vi "Main_capacitor-load.vi"(8 "error in":errorcluster) -> (0 "error out":errorcluster)   [LabVIEW 2019]
uses:
  _ctrl/create-rw-close.ctl
  Register/q-action_reg.ctl
  _ctrl/init-r-stop.ctl
  _ctrl/BP4610_cmd.ctl
  _ctrl/rw.ctl
  _ctrl/DSP_action.ctl
  _ctrl/Testing-info.ctl
  _ctrl/TestType.ctl
  ref_cap_ctrl-ref.ctl
  _ctrl/start.ctl
  common/Global 1.vi
  Devices/NI Board/cDAQ-9476 DO/cnt_Relay.ctl
  Devices/NI Board/cDAQ-9476 DO/cnt_do.ctl
  Devices/NI Board/cDAQ-9269 AO/type_signal.ctl
  Devices/NI Board/cDAQ-9269 AO/AO_q-data.ctl
  sequence_single.ctl
  SubVIs/common/Sample Check.ctl
  Data_cap.ctl
  cap_config.ctl
  Breakdown-Spec.ctl
  _ctrl/Error list.ctl
  _ctrl/DL950_config.ctl
  _ctrl/cDAQ-9269 Config.ctl
  Devices/NI Board/cDAQ-9269 AO/Set_AO_Wave-config.ctl
  Devices/NI Board/cDAQ-9221 AI/Set_NIAI.ctl
  _ctrl/BP4610_config.ctl
  _ctrl/DSP_config.ctl
panel:
  in  "수동_dl950":bool
  in  "수동_6":bool
  out "read_dl950":string
  out "error cluster 2":T1
  in  "Tab main":T2
  out "Relay6 result":T3
  out "Relay5 result":T3
  out "Relay4 result":T3
  out "Relay3 result":T3
  out "Relay2 result":T3
  out "Relay1 result":T3
  out "Graph 6":dbl[](graph)
  out "Graph 5":dbl[](graph)
  out "Graph 4":dbl[](graph)
  out "Graph 3":dbl[](graph)
  out "Graph 2":dbl[](graph)
  out "Graph 1":dbl[](graph)
  out "현재 채널":u8
  out "진행율_채널 %":u8(slide) scale=0.0..100.0
  out "진행율_전체 %":u8(slide) scale=0.0..100.0
  in  "파일 생성 주기[N]":dbl
  in  "저장 경로":path
  in  "시험명":string
  in  "CapTestSpec":T5 {"출력단 특성전류 Irms[mA]  Min" format="%#.2f"; "출력단 특성 전류 Irms[mA]  Max" format="%#.2f"; "출력단 단선 Irms[mA](이하)" format="%#.2f"; "제어단 특성 전류 Irms[mA] Min" format="%#.2f"; "제어단 특성 전류 Irms[mA] Max" format="%#.2f"; "제어단 단선 Irms[mA](이하)" format="%#.2f"}
  in  "CapTestConfig":T6={"출력전압[V]"=0.0, "출력전류[A]"=0.0, "방전 기준[V]"=0.0, "Freq"=0.0, "level[V]"=0.0, "duty"=0.0, "On time[ms]"=0.0, "Record Len"=4, "Time Div"=7, "Repeate"=1, "Test Cycle"=1, "OVP Level"=0.0, "OCP Level"=0.0, "Voltage+[V]"=20.0, "Current+[A]"=5.0, "Voltage-[V]"=-20.0, "Current-[A]"=-5.0} {"Current-[A]" min=-20.0 max=20.0 step=0.001; "Voltage-[V]" min=-115.0 max=115.0 step=0.01; "Current+[A]" min=0.0 max=60.0 step=0.01; "Voltage+[V]" min=0.0 max=120.0 step=0.1; "OCP Level" format="%#_13g"; "OVP Level" format="%#_13g"; "Time Div" items=["10m", "20ms", "50ms", "100ms", "200ms", "500ms", "1s", "2s"]; "Record Len" items=["10k", "25k", "50k", "100k", "250k", "500k", "1M", "2.5M", "5M", "10M", "25M", "50M", "100M", "250M", "500M", "1G", "2G", "4G", "5G", "10G", "20G", "50G"]}
  in  "Tab device":T7(tab)
  in  "DL950_config":T8={"Timeout"=10000, "Time Div"=19, "Acq Mode"=0, "Record Len"=5, "Record Num"=0, "Start Point"=0, "End Poin"=60000, "Visa"="TCPIP0::192.168.0.100::inst0::INSTR", "Config Voltage"=[{"Enable"=TRUE, "Ch"=0, "V Div"=12, "Coupling"=1, "Probe"=3, "Act.Items"=FALSE, "items"=[]}, {"Enable"=TRUE, "Ch"=0, "V Div"=12, "Coupling"=1, "Probe"=3, "Act.Items"=FALSE, "items"=[]}], "Trigger on"=FALSE, "Trigger Level"=0.0, "Reset"=FALSE, "Config Temp"=[], "Trig Mode"=1, "Trig Pos"=50.0, "Trigger Slope"=0, "Trigger Source "=1, "Trig Start -5"=-5.0, "End 5"=5.0} {"End 5" format="%.2g"; "Trig Start -5" format="%.2f"; "Trigger Source" items=["", "CH1", "CH2", "CH3", "CH4", "CH5", "CH6", "CH7", "CH8", "CH9", "CH10", "CH11", "CH12", "CH13", "CH14", "CH15", "CH16", "RMATH1", "RMATH2", "RMATH3", "RMATH4", "RMATH5", "RMATH6", "RMATH7", "RMATH8", "RMATH9", "RMATH10", "RMATH11", "RMATH12", "RMATH13", "RMATH14", "RMATH15", "RMATH16"]; "Trigger Slope" items=["Rising", "Falling", "Both"]; "Trig Pos" format="%.1f"; "Trig Mode" items=["Normal", "Auto", "Auto Level", "Single", "Single(N)", "On Start", "No Set"]; "Config Temp"."Type" items=["K", "E", "J", "T", "L", "U", "N", "R", "S", "B", "W", "Au7fe"]; "Config Temp"."Channel" items=["", "CH1", "CH2", "CH3", "CH4", "CH5", "CH6", "CH7", "CH8", "CH9", "CH10", "CH11", "CH12", "CH13", "CH14", "CH15", "CH16"]; "Trigger Level" format="%.3p"; "Config Voltage"."items" items=["Peak to Peak", "Amplitude", "Max", "Min", "High", "Low", "Average", "Middle", "Rms", "Standard Deviation", "+Overshoot", "-Overshoot", "Rise", "Fall", "Frequency", "Period", "+Width", "-Width", "Duty Cycle", "Pulse Count", "Burst1 Width", "Burst2 Width", "Average Frequency", "Average Period", "Int1TY", "Int2TY"]; "Config Voltage"."Probe" items=["1:1", "2:1", "5:1", "10:1", "20:1", "50:1", "100:1", "200:1", "500:1", "1000:1", "2000:1", "5000:1", "10k:1", "20k:1", "50k:1", "0.1A:1V", "0.2A:1V", "0.5A:1V", "1A:1V", "2A:1V", "5A:1V", "10A:1V", "20A:1V", "50A:1V", "100A:1V", "200A:1V", "250A:1V", "400A:1V", "500A:1V", "1kA:1V", "2kA:1V", "5kA:1V", "10kA:1V", "20kA:1V", "50kA:1V", "NoSet"]; "Config Voltage"."Ch" items=["None", "CH1", "CH2", "CH3", "CH4", "CH5", "CH6", "CH7", "CH8", "CH9", "CH10", "CH11", "CH12", "CH13", "CH14", "CH15", "CH16", "MATH1", "MATH2", "MATH3", "MATH4", "MATH5", "MATH6", "MATH7", "MATH8", "EVENT"]; "Config Voltage"."Coupling" items=["AC", "DC", "Ground", "AC-RMS", "DC-RMS"]; "Config Voltage"."V Div" items=["0.1m", "0.2m", "0.5m", "1m", "2m", "5m", "10m", "20m", "50m", "100m", "200m", "500m", "1", "2", "4", "5", "8", "10", "20", "40", "50", "80", "100", "200", "400", "500", "800", "1k", "2k", "4k", "5k", "8k", "10k", "20k", "25k", "50k", "100k", "250k", "500k", "1000k"]; "Record Len" items=["10k", "25k", "50k", "100k", "250k", "500k", "1M", "2.5M", "5M", "10M", "25M", "50M", "100M", "250M", "500M", "1G", "2G", "4G", "5G", "10G", "20G", "50G"]; "Acq Mode" items=["Normal", "Average", "Envelope"]; "Time Div" items=["100ns", "200ns", "500ns", "1us", "2us", "5us", "10us", "20us", "50us", "100us", "200us", "500us", "1ms", "2ms", "5ms", "10ms", "20ms", "50ms", "100ms", "200ms", "500ms", "1s", "2s", "3s", "4s", "5s", "6s", "10s", "20s", "30s", "1min", "2min", "3min", "4min", "5min", "6min", "10min", "12min", "30min", "1hour", "2hour", "3hour", "4hour", "5hour", "6hour", "8hour", "10hour", "12hour", "1day", "2day", "3day", "4day", "5day"]}
  in  "BP4610 Config":T9={"VISA"="", "Limit-BP"={"Set"=enum."Current", "Voltage+[V]"=20.0, "Current+[A]"=5.0, "Voltage-[V]"=-20.0, "Current-[A]"=-5.0}, "SET BP"={"Set"=enum."FREQ/WAVE", "Operation mode"=0, "Voltage[Vp-p]"=0.0, "Current[Ap-p]"=0.0, "Voltage[V]"=0.0, "Current[A]"=0.0, "Frequency[Hz]"=1.0, "Waveform"=enum."Sine"}} {"SET BP"."Frequency[Hz]" min=1.0 max=100000.0 step=0.1; "SET BP"."Current[A]" min=-20.0 max=20.0 step=0.001; "SET BP"."Voltage[V]" min=-115.0 max=115.0 step=0.01; "SET BP"."Current[Ap-p]" min=0.0 max=60.0 step=0.01; "SET BP"."Voltage[Vp-p]" min=0.0 max=120.0 step=0.1; "SET BP"."Operation mode" items=["CV-INT", "CV-EXT", "CV-ADD", "CC-INT", "CC-EXT", "CC-ADD"]; "Limit-BP"."Current-[A]" min=-20.0 max=20.0 step=0.001; "Limit-BP"."Voltage-[V]" min=-115.0 max=115.0 step=0.01; "Limit-BP"."Current+[A]" min=0.0 max=60.0 step=0.01; "Limit-BP"."Voltage+[V]" min=0.0 max=120.0 step=0.1}
  in  "DSP1950 Config":T10={"Port"="TCPIP0::192.168.0.14::HISLIP0::INSTR", "OVP Level"=0.0, "OCP Level"=0.0, "Current"=0.0, "Voltage"=0.0} {"OCP Level" format="%#_13g"; "OVP Level" format="%#_13g"}
  in  "cDAQ-9467 Config":tag
  in  "cDAQ 9221 Config":T11={"input terminal"=10083, "minimum value"=-60.0, "maximum value"=60.0, "number of samples"=1000, "rate"=10000.0, "sample mode"=10123, "physical channels"=""} {"sample mode" items=["Finite Samples"=10178, "Continuous Samples"=10123, "Hardware Timed Single Point"=12522]; "rate" format="%0.2f"; "maximum value" format="%^.2e"; "minimum value" format="%^.2e"; "input terminal" items=["default"=-1, "RSE"=10083, "NRSE"=10078, "Differential"=10106, "Pseudodifferential"=12529]}
  in  "AO_Wave-config":T12
  in  "cDAQ 9269 AO config":T13={"Ch"="cDAQ1Mod1/ao0", "Max V"=5.0, "Min V"=-5.0, " Rate"=1000.0, "N pts"=100, "sample mode"=10178} {"sample mode" items=["유한 샘플"=10178, "연속 샘플"=10123, "하드웨어 타이밍에 의한 단일 포인트"=12522]}
  in  "Graph":bool
  in  "Main":bool
  in  "TestStop":bool
  in  "TestStart":bool
  in  "TestReset":bool
  in  "Config":bool
  in  "Exit":bool
  # "Pre Charge Relay #2"
  # "Pre Charge Relay #5"
  # "제어단"
  # "출력단"
  # "온도기준"
  # "Control Power"
  # "Output Power"
  # "Oscilloscope"
  # "Discharge"
  # "Pre Charge Relay 내구시험 (캐패시터부하)"
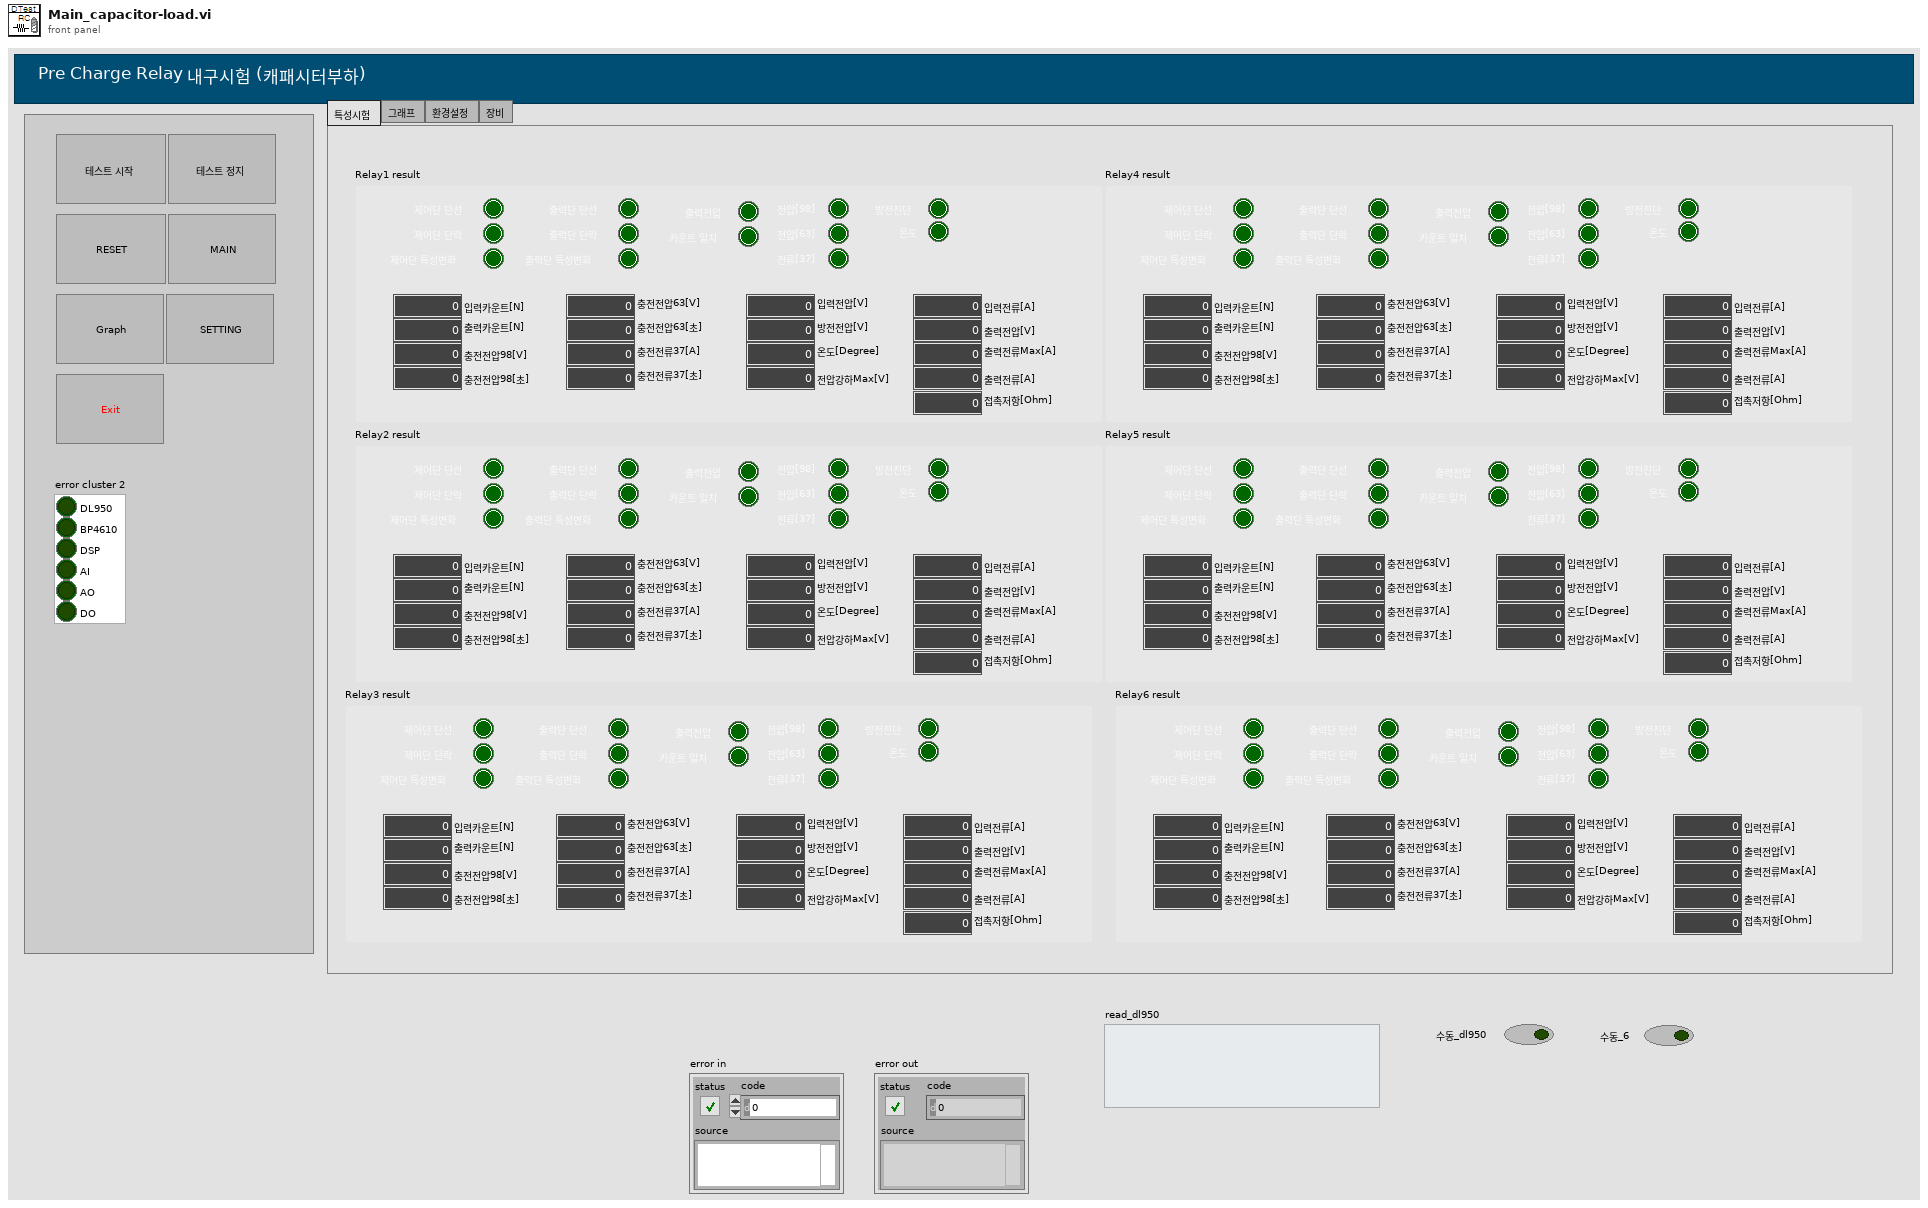
[diagram p1: front panel]
types:
  T1 = typedef "Error list.ctl" = cluster{"DL950":bool, "BP4610":bool, "DSP":bool, "AI":bool, "AO":bool, "DO":bool}
  T2 = typedef "Tap_내구시험.ctl" = enum32{"특성시험", "그래프", "환경설정", "장비"}
  T3 = typedef "Data_cap.ctl" = cluster{"입력카운트[N]":dbl, "출력카운트[N]":dbl, "입력전압[V]":dbl, "입력전류[A]":dbl, "출력전압[V]":dbl, "출력전류[A]":dbl, "충전전압98[V]":dbl, "충전전압63[V]":dbl, "충전전류37[A]":dbl, "방전전압[V]":dbl, "전압강하Max[V]":dbl, "출력전류Max[A]":dbl, "접촉저항[Ohm]":dbl, "충전전압98[초]":dbl, "충전전압63[초]":dbl, "충전전류37[초]":dbl, "제어단 단선":T4, "제어단 단락":T4, "제어단 특성변화":T4, "출력단 단선":T4, "출력단 단락":T4, "출력단 특성변화":T4, "카운트 일치":T4, "전압[98]":T4, "전압[63]":T4, "전류[37]":T4, "방전진단":T4, "출력전압":T4, "온도":T4, "온도[Degree]":dbl}
  T4 = typedef "Sample Check.ctl" = enum32{"idle", "OK", "NG", "Test"}
  T5 = typedef "Breakdown-Spec.ctl" = cluster{"제어단 단선 Irms[mA](이하)":dbl, "제어단 특성 전류 Irms[mA] Max":dbl, "제어단 특성 전류 Irms[mA] Min":dbl, "출력단 단선 Irms[mA](이하)":dbl, "출력단 특성 전류 Irms[mA]  Max":dbl, "출력단 특성전류 Irms[mA]  Min":dbl, "온도[degree]":dbl}
  T6 = typedef "cap_config.ctl" = cluster{"출력전압[V]":dbl, "출력전류[A]":dbl, "방전 기준[V]":dbl, "Freq":dbl, "level[V]":dbl, "duty":dbl, "On time[ms]":dbl, "Record Len":i32, "Time Div":u16, "Repeate":u32, "Test Cycle":u32, "OVP Level":dbl, "OCP Level":dbl, "Voltage+[V]":dbl, "Current+[A]":dbl, "Voltage-[V]":dbl, "Current-[A]":dbl}
  T7 = enum32{"DL950", "BP4610", "iDRC DSP1500", "cDAQ"}
  T8 = typedef "DL950_config.ctl" = cluster{"Timeout":u32, "Time Div":i32, "Acq Mode":i32, "Record Len":i32, "Record Num":i32, "Start Point":i64, "End Poin":i64, "Visa":refnum<visa-resource-name>, "Config Voltage":cluster{"Enable":bool, "Ch":u16, "V Div":i32, "Coupling":i32, "Probe":i32, "Act.Items":bool, "items":i32[]}[], "Trigger on":bool, "Trigger Level":dbl, "Reset":bool, "Config Temp":cluster{"Channel":u16, "Burn Out":bool, " Type ":i32}[], "Trig Mode":i32, "Trig Pos":dbl, "Trigger Slope":i32, "Trigger Source ":i32, "Trig Start -5":dbl, "End 5":dbl}
  T9 = typedef "BP4610_config.ctl" = cluster{"VISA":refnum<visa-resource-name>, "Limit-BP":cluster{"Set":enum16{"Current", "Voltage"}, "Voltage+[V]":dbl, "Current+[A]":dbl, "Voltage-[V]":dbl, "Current-[A]":dbl}, "SET BP":cluster{"Set":enum16{"Current", "Voltage", "FREQ/WAVE"}, "Operation mode":u16, "Voltage[Vp-p]":dbl, "Current[Ap-p]":dbl, "Voltage[V]":dbl, "Current[A]":dbl, "Frequency[Hz]":dbl, "Waveform":enum16{"Sine", "Square", "ARB 1", "ARB 2", "ARB 3", "ARB 4", "ARB 5", "ARB 6", "ARB 7", "ARB 8", "ARB 9", "ARB 10", "ARB 11", "ARB 12", "ARB 13", "ARB 14", "ARB 15", "ARB 16"}}}
  T10 = typedef "DSP_config.ctl" = cluster{"Port":refnum<visa-resource-name>, "OVP Level":dbl, "OCP Level":dbl, "Current":dbl, "Voltage":dbl}
  T11 = typedef "Set_NIAI.ctl" = cluster{"input terminal":i32, "minimum value":dbl, "maximum value":dbl, "number of samples":i32, "rate":dbl, "sample mode":i32, "physical channels":tag}
  T12 = typedef "Set_AO_Wave-config.ctl" = cluster{"offset":dbl, "Samples":i32, "duty":dbl, "Rate":dbl, "wfm":cluster{"Freq":dbl, "Amp":dbl, "Type":enum16{"Sine Wave", "Triangle Wave", "Square Wave", "Sawtooth Wave"}}}
  T13 = typedef "cDAQ-9269 Config.ctl" = cluster{"Ch":tag, "Max V":dbl, "Min V":dbl, " Rate":dbl, "N pts":i32, "sample mode":i32}
  T14 = typedef "cnt_do.ctl" = enum16{"open", "initial", "update", "run", "close"}
  T15 = typedef "init-r-stop.ctl" = enum16{"ini", "read", "stop"}
  T16 = typedef "create-rw-close.ctl" = enum16{"create", "write", "read", "delete", "close"}
  T17 = typedef "q-action_reg.ctl" = enum16{"Test-ini", "BP4610-on", "Pause", "Test-start", "Group-ini", "Ch-select", "Relay-on", "DSP-on", "DL950-start", "AO-start", "AO-delay", "Delay", "DL950-stop", "DSP-off", "Relay-off", "Ch-check", "UI-update", "Group-end", "Test-stop", "BP4610-off", "Test-finish", "Test-Manual", "DL950-Manual"}
  T18 = typedef "rw.ctl" = enum16{"read", "write"}
  T19 = typedef "ref_cap_ctrl-ref.ctl" = cluster{"cDAQ-9467 Config":refnum<vi>, "cDAQ 9221 Config":refnum<vi>, "cDAQ 9269 AO config":refnum<vi>, "AO_Wave-config":refnum<vi>, "TestSpec":refnum<vi>, "DL950_config":refnum<vi>, "BP4610 Config":refnum<vi>, "DSP1950 Config":refnum<vi>, "CapTest":refnum<vi>}
  T20 = enum16{"Config Save", "Config Load", "LastRUN Save", "LastRUN Load"}
  T21 = typedef "TestType.ctl" = enum16{"Manual", "Reg", "Cap", "B1", "B2", "B3"}
  T22 = typedef "BP4610_cmd.ctl" = enum16{"open", "read", "set", "set_seq", "limit", "limit_seq", "output on", "output off", "close"}
  T23 = typedef "DSP_action.ctl" = enum16{"False", "cont", "on", "off", "discont", "protection", "protection_seq", "preread", "level_seq", "level_m", "read", "stop", "exit"}
  T24 = typedef "Testing-info.ctl" = cluster{"전체채널수":u8, "현재채널번호":u8, "Irms":dbl, "입력전압":dbl, "입력전류":dbl, "출력전압":dbl, "출력전류":dbl, "온도":dbl, "제어단 단선":bool, "제어단 단락":bool, "제어단 특성변화":bool, "출력단 단선":bool, "출력단 단락":bool, "출력단 특성변화":bool, "출력단 전압":bool, "카운트 일치":bool, "Irms 판정":bool, "온도":bool, "테스트 회수":u32, "TestType":T25, "현재회수":u32, "Ch selection":cluster{"1ch":bool, "2ch":bool, "3ch":bool, "4ch":bool, "5ch":bool, "6ch":bool}, "반복":u32, "Path":path, "파일생성주기":u32, "start time":dbl, "stop time":dbl, "현재반복회수":u32, "NG":cluster{"입출력 카운트":bool, "출력전류RMS":bool}}
  T25 = typedef "sequence_single.ctl" = enum16{"Register", "RC", "B1", "B2", "B3"}
  T26 = typedef "system-status_내구.ctl" = enum16{"Initial", "Update", "Clear"}
  T27 = typedef "DSP_action.ctl" = enum16{"False", "cont", "on", "off", "discont", "protection", "preread", "level", "read", "stop", "exit"}
  T28 = typedef "start.ctl" = enum16{"init", "open", "set", "start", "stop", "read", "read_items", "query", "close", "T_single", "reset", "exit"}
  T29 = typedef "AO_q-data.ctl" = enum16{"init", "AO start"}
  T30 = typedef "cnt_Relay.ctl" = enum32{"R_Load", "R_out1", "R_out2", "R_out3", "R_out4", "R_out5", "R_out6", "R8", "R9", "R10", "R11", "R12", "R13", "R14", "R15", "R16", "R_in1", "R_in2", "R_in3", "R_in4", "R_in5", "R_in6", "R23", "R24", "R25", "R26", "R27", "R_red", "R_yellow", "R_green", "R_buz", "R_purple"}
  T31 = typedef "type_signal.ctl" = enum16{"wave", "level"}
  T32 = cluster{"1ch":bool, "2ch":bool, "3ch":bool, "4ch":bool, "5ch":bool, "6ch":bool}
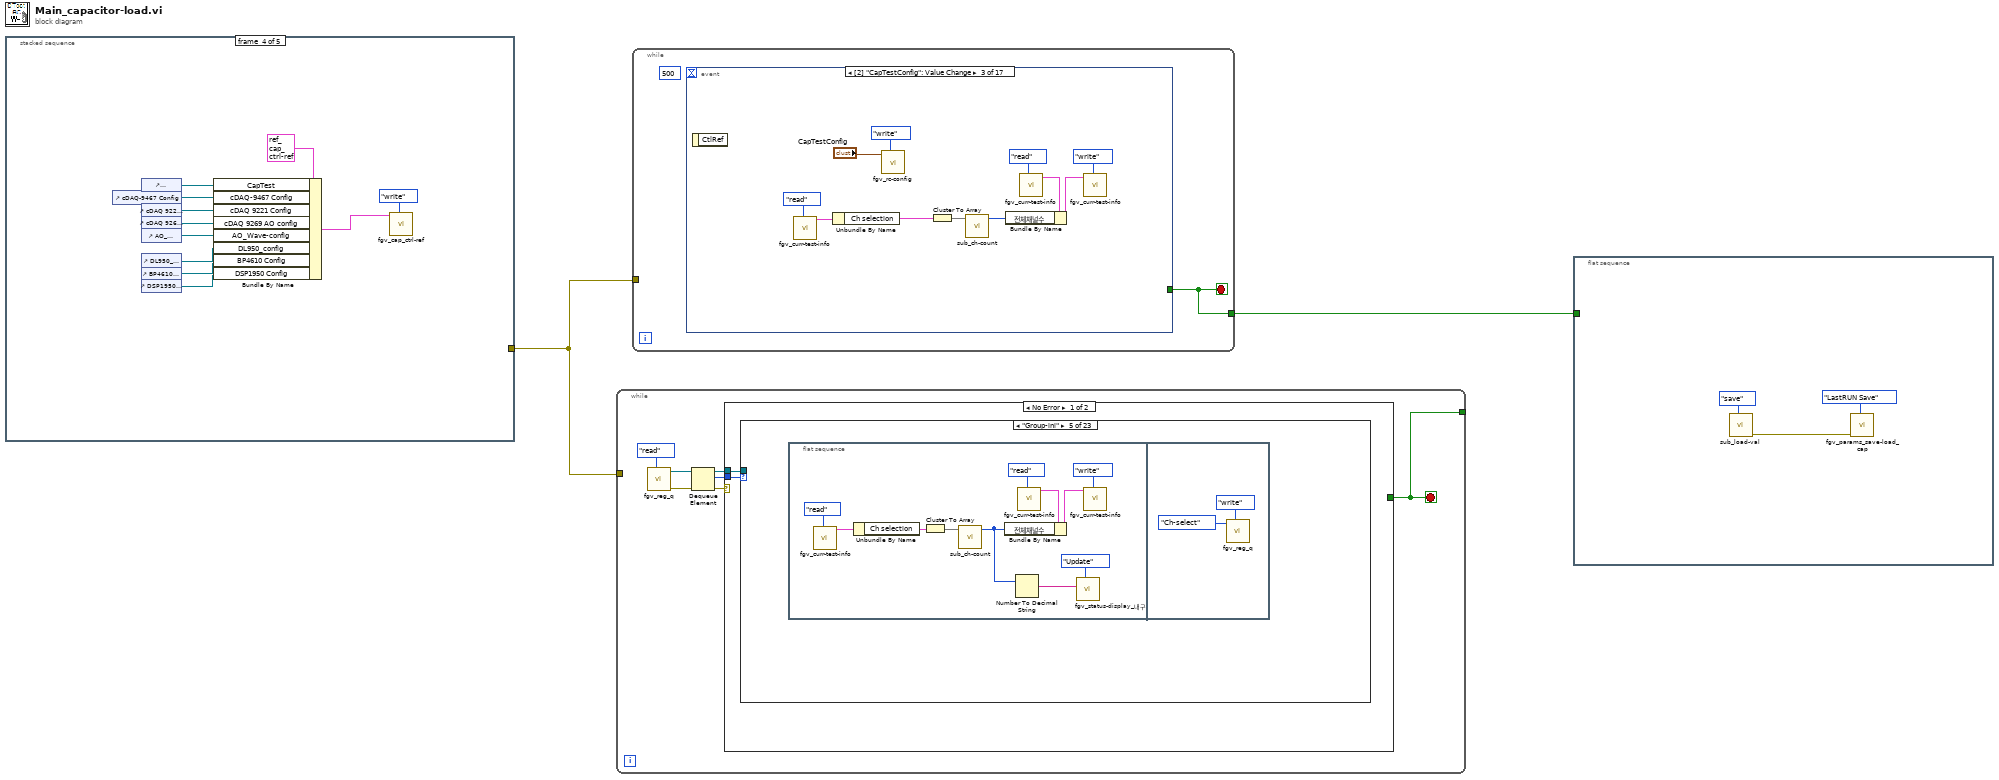
[diagram p0: block diagram]
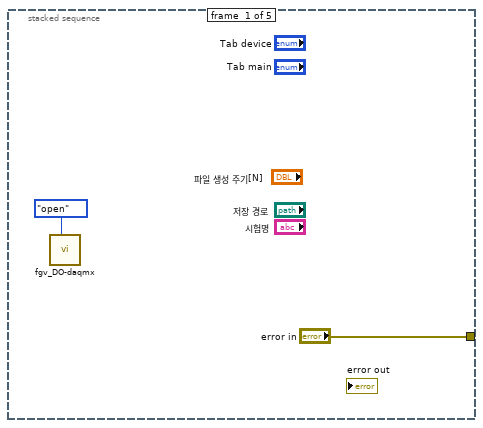
[diagram p2: hidden frame]
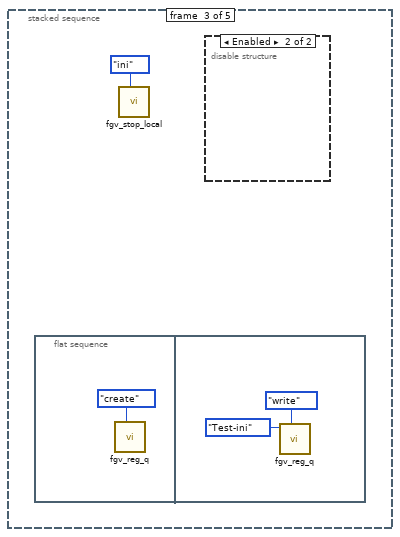
[diagram p4: hidden frame]
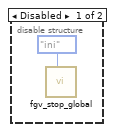
[diagram p5: hidden frame]
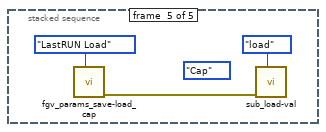
[diagram p6: hidden frame]
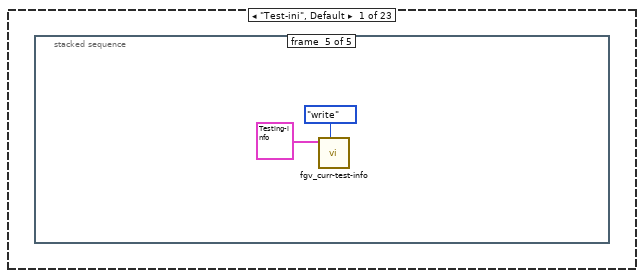
[diagram p7: hidden frame]
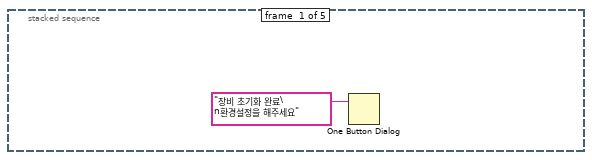
[diagram p8: hidden frame]
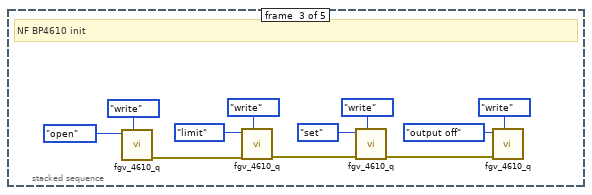
[diagram p10: hidden frame]
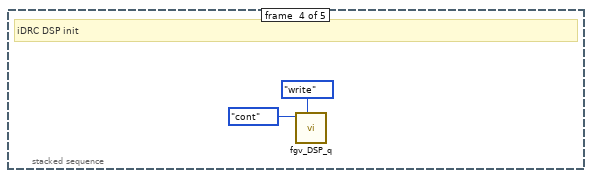
[diagram p11: hidden frame]
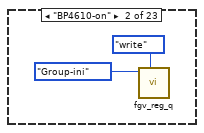
[diagram p12: hidden frame]
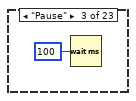
[diagram p13: hidden frame]
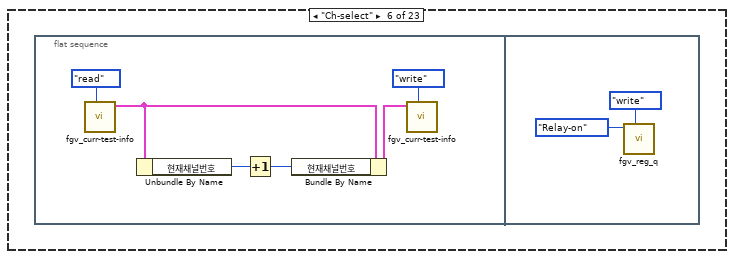
[diagram p15: hidden frame]
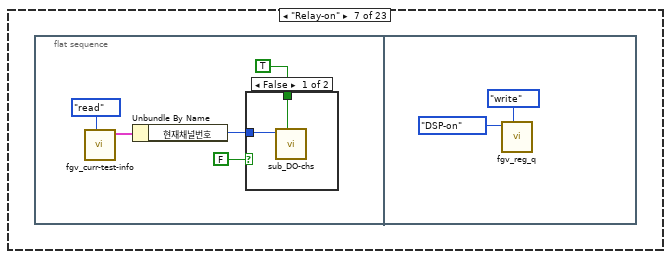
[diagram p16: hidden frame]
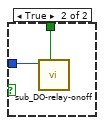
[diagram p17: hidden frame]
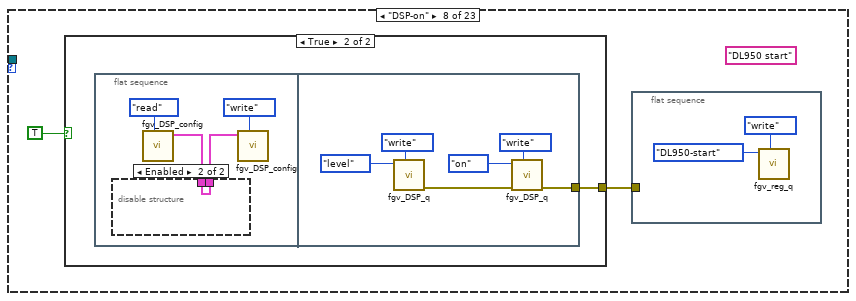
[diagram p18: hidden frame]
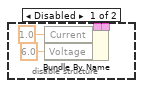
[diagram p20: hidden frame]
diagram:
  n1 = stacked-sequence {
    tunnel: ["error in" _ _ _ _] -> w2
    frame #0 {
      n2 = call "fgv_DO-daqmx.vi"("cnt"=cnt_do."open") -> ()  [unwired: 10 in, 1 out]
    }
    frame #1 {
    }
    frame #2 {
      n3 = flat-sequence {
        frame #0 {
          n4 = call "fgv_reg_q.vi"("cmd"=create-rw-close."create") -> ()  [unwired: 9 in, 2 out]
        }
        frame #1 {
          n5 = call "fgv_reg_q.vi"("cmd"=create-rw-close."write", "action"=q-action_reg."Test-ini") -> ()  [unwired: 8 in, 2 out]
        }
      }
      n6 = call "fgv_stop_local.vi"("cmd"=init-r-stop."ini") -> ()  [unwired: 9 in, 2 out]
      n7 = disable-structure shown="Enabled" {
        frame Disabled {
          n8 = call "fgv_stop_global.vi"("cmd"=init-r-stop."ini") -> ()  [unwired: 10 in, 1 out]
        }
        frame Enabled {
        }
      }
    }
    frame #3 {
      n9 = control-ref of="cDAQ-9467 Config"() -> (w19:refnum<vi>)
      n10 = control-ref of="CapTestConfig"() -> (w20:refnum<vi>)
      n11 = control-ref of="cDAQ 9221 Config"() -> (w18:refnum<vi>)
      n12 = control-ref of="cDAQ 9269 AO config"() -> (w17:refnum<vi>)
      n13 = control-ref of="AO_Wave-config"() -> (w16:refnum<vi>)
      n14 = control-ref of="DL950_config"() -> (w12:refnum<vi>)
      n15 = control-ref of="BP4610 Config"() -> (w11:refnum<vi>)
      n16 = control-ref of="DSP1950 Config"() -> (w10:refnum<vi>)
      n17 = Bundle By Name(cluster=T19 {"cDAQ-9467 Config"=refnum, "cDAQ 9221 Config"=refnum, "cDAQ 9269 AO config"=refnum, "AO_Wave-config"=refnum, "TestSpec"=refnum, "DL950_config"=refnum, "BP4610 Config"=refnum, "DSP1950 Config"=refnum, "CapTest"=refnum} ("input cluster"), "CapTest"=w20, "cDAQ-9467 Config"=w19, "cDAQ 9221 Config"=w18, "cDAQ 9269 AO config"=w17, "AO_Wave-config"=w16, "DL950_config"=w12, "BP4610 Config"=w11, "DSP1950 Config"=w10) -> (w14:T19)
      n18 = call "fgv_cap_ctrl-ref.vi"("cmd"=rw."write", "input cluster"=w14) -> ()  [unwired: 9 in, 1 out]
    }
    frame #4 {
      (unwired) TestType."Cap" ("TestType")
      n19 = call "fgv_params_save-load_cap.vi"("cmd"=T20."LastRUN Load") -> ("error out"=w21:errorcluster)  [unwired: 9 in, 1 out]
      n20 = call "sub_load-val.vi"("cmd"=enum16{"load", "save"}."load", "Error in"=w21) -> ()  [unwired: 9 in, 1 out]
    }
  }
  n21 = while {
    tunnel: w2 -> [_]
    tunnel: [w25] -> _
    stop <- w25 stop-if-true
    n22 = call "fgv_reg_q.vi"("cmd"=create-rw-close."read") -> ("error out"=w26:errorcluster, "queue out"=w27:refnum<queue>)  [unwired: 9 in]
    n23 = Dequeue Element(queue=w27, error in (no error)=w26) -> (queue out=w24:refnum<queue>, element=w29:T17, error out=w30:errorcluster)  [unwired: 1 in, 1 out]
    n24 = case shown="No Error" w30 {
      tunnel: w29 -> [w32 _]
      tunnel: [_ TRUE] -> w25
      tunnel: w24 -> [w31 _]
      frame No Error {
        n25 = case shown="\"Group-ini\"" w32 {
          tunnel: w31 -> [_ _ _ _ _ _ _ _ _ _ _ _ _ _ _ _ _ _ w169 _ _ _ _]
          frame "Test-ini", Default {
            n26 = stacked-sequence {
              frame #0 {
                n27 = One Button Dialog(message="장비 초기화 완료\n환경설정을 해주세요" ("메시지")) -> ()  [unwired: 1 in, 1 out]
              }
              frame #1 {
                # "UI 초기화"
              }
              frame #2 {
                # "NF BP4610 init"
                n28 = call "fgv_4610_q.vi"("cmd"=create-rw-close."write", "action"=BP4610_cmd."open") -> ("error out"=w40:errorcluster)  [unwired: 8 in, 1 out]
                n29 = call "fgv_4610_q.vi"("cmd"=create-rw-close."write", "error in"=w40, "action"=BP4610_cmd."limit") -> ("error out"=w35:errorcluster)  [unwired: 7 in, 1 out]
                n30 = call "fgv_4610_q.vi"("cmd"=create-rw-close."write", "error in"=w35, "action"=BP4610_cmd."set") -> ("error out"=w34:errorcluster)  [unwired: 7 in, 1 out]
                n31 = call "fgv_4610_q.vi"("cmd"=create-rw-close."write", "error in"=w34, "action"=BP4610_cmd."output off") -> ()  [unwired: 7 in, 2 out]
              }
              frame #3 {
                # "iDRC DSP init"
                n32 = call "fgv_DSP_q.vi"("cmd"=create-rw-close."write", "action"=DSP_action."cont") -> ()  [unwired: 8 in, 2 out]
              }
              frame #4 {
                n33 = call "fgv_curr-test-info.vi"("cmd"=rw."write", "현재테스트 정보"=T24 {"전체채널수"=0, "현재채널번호"=0, "Irms"=0.0, "입력전압"=0.0, "입력전류"=0.0, "출력전압"=0.0, "출력전류"=0.0, "온도"=0.0, "제어단 단선"=FALSE, "제어단 단락"=FALSE, "제어단 특성변화"=FALSE, "출력단 단선"=FALSE, "출력단 단락"=FALSE, "출력단 특성변화"=FALSE, "출력단 전압"=FALSE, "카운트 일치"=FALSE, "Irms 판정"=FALSE, "온도"=FALSE, "테스트 회수"=0, "TestType"=enum."Register", "현재회수"=0, "Ch selection"={"1ch"=FALSE, "2ch"=FALSE, "3ch"=FALSE, "4ch"=FALSE, "5ch"=FALSE, "6ch"=FALSE}, "반복"=0, "Path"=path "", "파일생성주기"=0, "start time"=0.0, "stop time"=0.0, "현재반복회수"=0, "NG"={"입출력 카운트"=FALSE, "출력전류RMS"=FALSE}}) -> ()  [unwired: 9 in, 1 out]
              }
            }
          }
          frame "BP4610-on" {
            n34 = call "fgv_reg_q.vi"("cmd"=create-rw-close."write", "action"=q-action_reg."Group-ini") -> ()  [unwired: 8 in, 2 out]
          }
          frame "Pause" {
            n35 = Wait (ms)(milliseconds to wait=u32 100 ("대기 시간 (ms)")) -> ()  [unwired: 1 out]
          }
          frame "Test-start" {
          }
          frame "Group-ini" {
            n36 = flat-sequence {
              frame #0 {
                n37 = call "fgv_curr-test-info.vi"("cmd"=rw."read") -> ("현재테스트 정보 2"=w53:T24)  [unwired: 10 in]
                n38 = Unbundle By Name(w53) -> ("Ch selection"=w52:T32)
                n39 = Cluster To Array(cluster=w52) -> (array=w60:bool[])
                n40 = call "sub_ch-count.vi"("ch config"=w60) -> ("ch num"=w55:u8)  [unwired: 10 in]
                n41 = Number To Decimal String(number=w55) -> (decimal integer string=w56:string)  [unwired: 1 in]
                n42 = call "fgv_curr-test-info.vi"("cmd"=rw."read") -> ("현재테스트 정보 2"=w59:T24)  [unwired: 10 in]
                n43 = Bundle By Name(cluster=w59, "전체채널수"=w55) -> (w58:T24)
                n44 = call "fgv_status-display_내구.vi"("Mode"=system-status_내구."Update", "title"=w56) -> ()  [unwired: 9 in, 1 out]
                n45 = call "fgv_curr-test-info.vi"("cmd"=rw."write", "현재테스트 정보"=w58) -> ()  [unwired: 9 in, 1 out]
              }
              frame #1 {
                n46 = call "fgv_reg_q.vi"("cmd"=create-rw-close."write", "action"=q-action_reg."Ch-select") -> ()  [unwired: 8 in, 2 out]
              }
            }
          }
          frame "Ch-select" {
            n47 = flat-sequence {
              frame #0 {
                n48 = call "fgv_curr-test-info.vi"("cmd"=rw."read") -> ("현재테스트 정보 2"=w68:T24)  [unwired: 10 in]
                n49 = Unbundle By Name(w68) -> ("현재채널번호"=w66:u8)
                n50 = Increment(x=w66) -> (x+1=w65:u8)
                n51 = Bundle By Name(cluster=w68, "현재채널번호"=w65) -> (w67:T24)
                n52 = call "fgv_curr-test-info.vi"("cmd"=rw."write", "현재테스트 정보"=w67) -> ()  [unwired: 9 in, 1 out]
              }
              frame #1 {
                n53 = call "fgv_reg_q.vi"("cmd"=create-rw-close."write", "action"=q-action_reg."Relay-on") -> ()  [unwired: 8 in, 2 out]
              }
            }
          }
          frame "Relay-on" {
            n54 = flat-sequence {
              frame #0 {
                n55 = call "fgv_curr-test-info.vi"("cmd"=rw."read") -> ("현재테스트 정보 2"=w76:T24)  [unwired: 10 in]
                n56 = Unbundle By Name(w76) -> ("현재채널번호"=w75:u8)
                n57 = case shown="False" FALSE {
                  tunnel: w75 -> [w78 w81]
                  tunnel: TRUE ("onoff") -> [w79 w80]
                  frame False {
                    n58 = call "sub_DO-chs.vi"("onoff"=w79, "ch"=w78) -> ()  [unwired: 9 in, 1 out]
                  }
                  frame True {
                    n59 = call "sub_DO-relay-onoff.vi"("onoff"=w80, "현재채널번호"=w81) -> ()  [unwired: 10 in]
                  }
                }
              }
              frame #1 {
                n60 = call "fgv_reg_q.vi"("cmd"=create-rw-close."write", "action"=q-action_reg."DSP-on") -> ()  [unwired: 8 in, 2 out]
              }
            }
          }
          frame "DSP-on" {
            (unwired) "DL950 start"
            n61 = case shown="True" TRUE {
              tunnel: [_ w88] -> w84
              frame False {
              }
              frame True {
                n62 = flat-sequence {
                  tunnel: [w98] -> w88
                  frame #0 {
                    n63 = call "fgv_DSP_config.vi"("cmd"=rw."read") -> ("DSP1950 Config 2"=w92:T10)  [unwired: 9 in, 1 out]
                    n64 = disable-structure shown="Enabled" {
                      disable-tunnel: w92 -> [w96 w97]
                      disable-tunnel: [w95 w97] -> w91
                      frame Disabled {
                        n65 = Bundle By Name(cluster=w96, "Current"=1.0, "Voltage"=6.0) -> (w95:T10)
                      }
                      frame Enabled {
                      }
                    }
                    n66 = call "fgv_DSP_config.vi"("cmd"=rw."write", "DSP1950 Config"=w91) -> ()  [unwired: 8 in, 2 out]
                  }
                  frame #1 {
                    n67 = call "fgv_DSP_q.vi"("cmd"=create-rw-close."write", "action"=DSP_action."level") -> ("error out"=w99:errorcluster)  [unwired: 8 in, 1 out]
                    n68 = call "fgv_DSP_q.vi"("cmd"=create-rw-close."write", "error in"=w99, "action"=DSP_action."on") -> ("error out"=w98:errorcluster)  [unwired: 7 in, 1 out]
                  }
                }
              }
            }
            n69 = flat-sequence {
              tunnel: w84 -> [_]
              frame #0 {
                n70 = call "fgv_reg_q.vi"("cmd"=create-rw-close."write", "action"=q-action_reg."DL950-start") -> ()  [unwired: 8 in, 2 out]
              }
            }
          }
          frame "DL950-start" {
            n71 = flat-sequence {
              frame #0 {
                n72 = call "fgv_DL950_q.vi"("cmd"=create-rw-close."write", "data"=start."start") -> ()  [unwired: 8 in, 2 out]
              }
              frame #1 {
                n73 = Wait (ms)(milliseconds to wait=u32 1000 ("대기 시간 (ms)")) -> ()  [unwired: 1 out]
              }
              frame #2 {
                n74 = call "fgv_reg_q.vi"("cmd"=create-rw-close."write", "action"=q-action_reg."AO-start") -> ()  [unwired: 8 in, 2 out]
              }
            }
          }
          frame "AO-start" {
            n75 = call "fgv_AO_q.vi"("cmd"=create-rw-close."write", "data"=AO_q-data."AO start") -> ("error out"=w110:errorcluster)  [unwired: 8 in, 1 out]
            n76 = call "fgv_reg_q.vi"("cmd"=create-rw-close."write", "error in"=w110, "action"=q-action_reg."AO-delay") -> ()  [unwired: 7 in, 2 out]
          }
          frame "AO-delay" {
            n77 = Wait (ms)(milliseconds to wait=u32 100) -> ()  [unwired: 1 out]
            n78 = call "fgv_reg_q.vi"("cmd"=create-rw-close."write", "action"=q-action_reg."DL950-stop") -> ()  [unwired: 8 in, 2 out]
          }
          frame "Delay" {
          }
          frame "DL950-stop" {
            n79 = call "fgv_DL950_q.vi"("cmd"=create-rw-close."write", "data"=start."stop") -> ("error out"=w119:errorcluster)  [unwired: 8 in, 1 out]
            n80 = call "fgv_DL950_q.vi"("cmd"=create-rw-close."write", "error in"=w119, "data"=start."read") -> ()  [unwired: 7 in, 2 out]
            n81 = call "fgv_reg_q.vi"("cmd"=create-rw-close."write", "action"=q-action_reg."DSP-off") -> ()  [unwired: 8 in, 2 out]
          }
          frame "DSP-off" {
            n82 = flat-sequence {
              frame #0 {
                n83 = call "fgv_DSP_config.vi"("cmd"=rw."read") -> ("DSP1950 Config 2"=w127:T10)  [unwired: 9 in, 1 out]
                n84 = Bundle By Name(cluster=w127, "Voltage"=0.0, "Current"=0.0) -> (w126:T10)
                n85 = call "fgv_DSP_config.vi"("cmd"=rw."write", "DSP1950 Config"=w126) -> ()  [unwired: 8 in, 2 out]
              }
              frame #1 {
                n86 = call "fgv_DSP_visa.vi"("action"=DSP_action."level") -> ("error out"=w131:errorcluster)  [unwired: 10 in]
                n87 = call "fgv_DSP_visa.vi"("action"=DSP_action."on", "error in"=w131) -> ()  [unwired: 9 in, 1 out]
              }
              frame #2 {
                n88 = Wait (ms)(milliseconds to wait=u32 400 ("대기 시간 (ms)")) -> ()  [unwired: 1 out]
                n89 = call "fgv_reg_q.vi"("cmd"=create-rw-close."write", "action"=q-action_reg."Relay-off") -> ()  [unwired: 8 in, 2 out]
              }
            }
          }
          frame "Relay-off" {
            n90 = flat-sequence {
              frame #0 {
                n91 = call "fgv_curr-test-info.vi"("cmd"=rw."read") -> ("현재테스트 정보 2"=w138:T24)  [unwired: 10 in]
                n92 = Unbundle By Name(w138) -> ("현재채널번호"=w137:u8)
                n93 = call "sub_DO-relay-onoff.vi"("onoff"=FALSE, "현재채널번호"=w137) -> ()  [unwired: 10 in]
              }
              frame #1 {
                n94 = call "fgv_reg_q.vi"("cmd"=create-rw-close."write", "action"=q-action_reg."UI-update") -> ()  [unwired: 8 in, 2 out]
              }
            }
          }
          frame "Ch-check" {
            n95 = call "fgv_curr-test-info.vi"("cmd"=rw."read") -> ("현재테스트 정보 2"=w150:T24)  [unwired: 10 in]
            n96 = Unbundle By Name(w150) -> ("전체채널수"=w148:u8, "현재채널번호"=w147:u8)
            n97 = Equal?(x=w148, y=w147) -> (x = y?=w146:bool)
            n98 = case shown="True" w146 {
              frame False {
              }
              frame True {
                n99 = call "fgv_curr-test-info.vi"("cmd"=rw."read") -> ("현재테스트 정보 2"=w153:T24)  [unwired: 10 in]
                n100 = Unbundle By Name(w153) -> ("테스트 회수"=w152:u32)
                n101 = Increment(x=w152) -> (x+1=w151:u32)
                n102 = Bundle By Name(cluster=w153, "현재채널번호"=u8 0, "테스트 회수"=w151) -> (w155:T24)
                n103 = call "fgv_curr-test-info.vi"("cmd"=rw."write", "현재테스트 정보"=w155) -> ()  [unwired: 9 in, 1 out]
              }
            }
            n104 = Select(t=q-action_reg."Group-end" ("action"), s=w146, f=q-action_reg."Ch-select" ("action")) -> (s? t:f=w142:T17)
            n105 = call "fgv_reg_q.vi"("cmd"=create-rw-close."write", "action"=w142) -> ()  [unwired: 8 in, 2 out]
          }
          frame "UI-update" {
          }
          frame "Group-end" {
            n106 = call "fgv_curr-test-info.vi"("cmd"=rw."read") -> ("현재테스트 정보 2"=w165:T24)  [unwired: 10 in]
            n107 = Unbundle By Name(w165) -> ("현재회수"=w158:u32, "테스트 회수"=w164:u32)
            n108 = Equal?(x=w158, y=w164) -> (x = y?=w163:bool)
            n109 = Select(t=q-action_reg."BP4610-off" ("action"), s=w163, f=q-action_reg."Group-ini" ("action")) -> (s? t:f=w159:T17)
            n110 = Select(t="테스트종료", s=w163, f="그룹초기화") -> ()  [unwired: 1 out]
            n111 = call "fgv_reg_q.vi"("cmd"=create-rw-close."write", "action"=w159) -> ()  [unwired: 8 in, 2 out]
          }
          frame "Test-stop" {
            n112 = Flush Queue(queue=w169) -> ()  [unwired: 1 in, 3 out]
            n113 = flat-sequence {
              frame #0 {
                n114 = for {
                  N: 6 -> [_]
                  tunnel: FALSE ("onoff") -> [w172]
                  i -> [w174]
                  n115 = Increment(x=w174) -> (x+1=w173:i32)
                  n116 = call "sub_DO-relay-onoff.vi"("onoff"=w172, "현재채널번호"=w173) -> ()  [unwired: 10 in]
                }
              }
              frame #1 {
                n117 = call "fgv_reg_q.vi"("cmd"=create-rw-close."write", "action"=q-action_reg."Test-finish") -> ()  [unwired: 8 in, 2 out]
              }
            }
          }
          frame "BP4610-off" {
            n118 = flat-sequence {
              frame #0 {
                n119 = call "fgv_4610_q.vi"("cmd"=create-rw-close."write", "action"=BP4610_cmd."output off") -> ()  [unwired: 8 in, 2 out]
              }
              frame #1 {
                n120 = call "fgv_reg_q.vi"("cmd"=create-rw-close."write", "action"=q-action_reg."Test-stop") -> ()  [unwired: 8 in, 2 out]
              }
            }
          }
          frame "Test-finish" {
            n121 = One Button Dialog(message="테스트 완료" ("메시지")) -> ()  [unwired: 1 in, 1 out]
            n122 = flat-sequence {
              frame #0 {
                n123 = call "fgv_curr-test-info.vi"("cmd"=rw."read") -> ("현재테스트 정보 2"=w182:T24)  [unwired: 10 in]
                n124 = Bundle By Name(cluster=w182, "현재채널번호"=u8 0) -> (w184:T24)
                n125 = call "fgv_curr-test-info.vi"("cmd"=rw."write", "현재테스트 정보"=w184) -> ()  [unwired: 9 in, 1 out]
              }
              frame #1 {
              }
            }
          }
          frame "Test-Manual" {
            n126 = stacked-sequence {
              frame #0 {
                n127 = for {
                  tunnel: cluster{"Relay":T30, "Boolean":bool}[] [{"Relay"=enum."R_in1", "Boolean"=TRUE}, {"Relay"=enum."R_out1", "Boolean"=TRUE}] -> [w188] mode=indexing
                  n128 = flat-sequence {
                    tunnel: w188 -> [w189]
                    frame #0 {
                      n129 = global write "Global 1.vi" "Relay"(w189) -> ()
                    }
                    frame #1 {
                      n130 = call "fgv_DO-daqmx.vi"("cnt"=cnt_do."update") -> ()  [unwired: 10 in, 1 out]
                    }
                  }
                }
              }
              frame #1 {
                n131 = call "fgv_DO_q.vi"("cmd"=create-rw-close."write", "data"=start."start") -> ()  [unwired: 8 in, 2 out]
              }
              frame #2 {
                n132 = call "fgv_DL950_q.vi"("cmd"=create-rw-close."write", "data"=start."T_single") -> ()  [unwired: 8 in, 2 out]
              }
              frame #3 {
                n133 = call "fgv_4610_q.vi"("cmd"=create-rw-close."write", "action"=BP4610_cmd."limit") -> ("error out"=w198:errorcluster)  [unwired: 8 in, 1 out]
                n134 = call "fgv_4610_q.vi"("cmd"=create-rw-close."write", "error in"=w198, "action"=BP4610_cmd."set") -> ("error out"=w195:errorcluster)  [unwired: 7 in, 1 out]
                n135 = call "fgv_4610_q.vi"("cmd"=create-rw-close."write", "error in"=w195, "action"=BP4610_cmd."output on") -> ()  [unwired: 7 in, 2 out]
              }
              frame #4 {
                n136 = call "fgv_DSP_q.vi"("cmd"=create-rw-close."write", "action"=DSP_action."level") -> ("error out"=w203:errorcluster)  [unwired: 8 in, 1 out]
                n137 = call "fgv_DSP_q.vi"("cmd"=create-rw-close."write", "error in"=w203, "action"=DSP_action."on") -> ()  [unwired: 7 in, 2 out]
              }
              frame #5 {
                n138 = Wait (ms)(milliseconds to wait=u32 500) -> ()  [unwired: 1 out]
              }
              frame #6 {
                n139 = call "fgv_AO_wave-config.vi"("cmd"=rw."read") -> ("Square Wave 2"=w212:T12)  [unwired: 10 in]
                n140 = Bundle By Name(cluster=w212, "wfm.Amp"=12.0 ("Waveform.Amplitude")) -> (w211:T12)
                n141 = call "signalGenerator.vi"("cnt"=type_signal."level", "Square Wave"=w211) -> ("error out"=w216:errorcluster)  [unwired: 8 in, 1 out]
                n142 = call "fgv_AO_q.vi"("cmd"=create-rw-close."write", "error in"=w216, "data"=AO_q-data."AO start") -> ()  [unwired: 7 in, 2 out]
              }
              frame #7 {
                # "0.2초 온"
                n143 = Wait (ms)(milliseconds to wait=u32 200) -> ()  [unwired: 1 out]
              }
              frame #8 {
                n144 = call "fgv_AO_wave-config.vi"("cmd"=rw."read") -> ("Square Wave 2"=w221:T12)  [unwired: 10 in]
                n145 = Bundle By Name(cluster=w221, "wfm.Amp"=0.0 ("Waveform.Amplitude")) -> (w220:T12)
                n146 = call "signalGenerator.vi"("cnt"=type_signal."level", "Square Wave"=w220) -> ("error out"=w225:errorcluster)  [unwired: 8 in, 1 out]
                n147 = call "fgv_AO_q.vi"("cmd"=create-rw-close."write", "error in"=w225, "data"=AO_q-data."AO start") -> ()  [unwired: 7 in, 2 out]
              }
              frame #9 {
                n148 = call "fgv_4610_q.vi"("cmd"=create-rw-close."write", "action"=BP4610_cmd."output off") -> ()  [unwired: 8 in, 2 out]
              }
              frame #10 {
                n149 = Wait (ms)(milliseconds to wait=u32 200) -> ()  [unwired: 1 out]
                n150 = global write "Global 1.vi" "String"("MEASURE:CHANNEL2:RISE:VALUE?\n:MEASURE:CHANNEL6:FALL:VALUE?\n:MEASURE:CHANNEL2:DPROXIMAL:PERCENT 0,50,98\n:MEASURE:TRANGE -5,5\n:MEASURE:CHANNEL2:RMS:VALUE?\n:MEASURE:CHANNEL3:MAXimum:VALUE?\n:MEASURE:CHANNEL4:MAXimum:VALUE?\n:MEASURE:CHANNEL6:RMS:VALUE?\n:MEASURE:TRANGE -4.2,0\n:MEASURE:CHANNEL2:RISE:VALUE?" ("String")) -> ()
              }
              frame #11 {
                n151 = call "fgv_DL950_q.vi"("cmd"=create-rw-close."write", "data"=start."query") -> ()  [unwired: 8 in, 2 out]
              }
              frame #12 {
                n152 = for {
                  tunnel: cluster{"Relay":T30, "Boolean":bool}[] [{"Relay"=enum."R_in1", "Boolean"=FALSE}, {"Relay"=enum."R_out1", "Boolean"=FALSE}] -> [w233] mode=indexing
                  n153 = global write "Global 1.vi" "Relay"(w233) -> ()
                }
              }
              frame #13 {
                n154 = call "fgv_DO_q.vi"("cmd"=create-rw-close."write", "data"=start."start") -> ()  [unwired: 8 in, 2 out]
                n155 = Wait (ms)(milliseconds to wait=u32 200) -> ()  [unwired: 1 out]
              }
              frame #14 {
                n156 = call "fgv_DSP_q.vi"("cmd"=create-rw-close."write", "action"=DSP_action."off") -> ()  [unwired: 8 in, 2 out]
              }
              frame #15 {
                n157 = for {
                  tunnel: cluster{"Relay":T30, "Boolean":bool}[] [{"Relay"=enum."R_Load", "Boolean"=TRUE}] -> [w240] mode=indexing
                  n158 = global write "Global 1.vi" "Relay"(w240) -> ()
                }
              }
              frame #16 {
                n159 = call "fgv_DO-daqmx.vi"("cnt"=cnt_do."update") -> ()  [unwired: 10 in, 1 out]
              }
              frame #17 {
                n160 = Wait (ms)(milliseconds to wait=u32 2000) -> ()  [unwired: 1 out]
              }
              frame #18 {
                n161 = call "fgv_DO_q.vi"("cmd"=create-rw-close."write", "data"=start."start") -> ()  [unwired: 8 in, 2 out]
              }
              frame #19 {
                n162 = global read "Global 1.vi" "read_dl950"() -> (→"read_dl950":string)
              }
            }
          }
          frame "DL950-Manual" {
            n163 = stacked-sequence {
              frame #0 {
                n164 = call "fgv_DL950_q.vi"("cmd"=create-rw-close."write", "data"=start."set") -> ()  [unwired: 8 in, 2 out]
              }
              frame #1 {
                n165 = global write "Global 1.vi" "String"(":MEASURE:TRANGE -5,5\n:MEASURE:CHANNEL2:RMS:STATE ON\n:MEASURE:CHANNEL2:RISE:STATE ON\n:MEASURE:CHANNEL3:MAXimum:STATE ON\n:MEASURE:CHANNEL4:MAXimum:STATE ON\n:MEASURE:CHANNEL5:RMS:STATE ON\n:MEASURE:CHANNEL6:RMS:STATE ON\n:MEASURE:CHANNEL6:FALL:STATE ON\n:MEASURE:CHANNEL2:DPROXIMAL:PERCENT 0,30,63\n:MEASURE:CHANNEL6:DPROXIMAL:PERCENT 37,50,100" ("String")) -> ()
              }
              frame #2 {
                n166 = call "fgv_DL950_q.vi"("cmd"=create-rw-close."write", "data"=start."query") -> ()  [unwired: 8 in, 2 out]
              }
            }
          }
        }
      }
      frame Error {
        # "Return true in any case that should stop the loop."
      }
    }
  }
  n167 = while {
    tunnel: w2 -> [_]
    tunnel: [w252] -> w1
    stop <- w252 stop-if-true
    (unwired) 500
    n168 = event shown="[2] \"CapTestConfig\": Value Change" {
      selector: _ -> [_ _ _ _ _ _ _ _ _ _ _ _ _ _ _ _ _]
      dyn-events: _ -> [_ _ _ _ _ _ _ _ _ _ _ _ _ _ _ _ _]
      timeout: _ -> [_ _ _ _ _ _ _ _ _ _ _ _ _ _ _ _ _]
      tunnel: [w253 _ _ _ _ _ _ _ _ _ _ _ _ _ _ _ _] -> w252
      event "Exit": Value Change {
        n169 = event-data() -> ()  [unwired: 1 in, 1 out]
        n170 = flat-sequence {
          tunnel: ["Exit"] -> w253
          frame #0 {
            n171 = call "fgv_4610_q.vi"("cmd"=create-rw-close."write", "action"=BP4610_cmd."output off") -> ()  [unwired: 8 in, 2 out]
            n172 = Wait (ms)(milliseconds to wait=u32 500) -> ()  [unwired: 1 out]
          }
          frame #1 {
            n173 = call "fgv_reg_q.vi"("cmd"=create-rw-close."close") -> ()  [unwired: 9 in, 2 out]
          }
        }
      }
      event "Config", "Main", "Graph": Value Change {
        n174 = event-data() -> ("CtlRef"=w261:refnum<vi>)  [unwired: 1 in]
        n175 = property class="Bool"(reference=w261) -> ("Label.Text"=w260:string)  [unwired: 1 in, 2 out]
        n176 = case shown="\"Main\"" w260 {
          tunnel: [Tap_내구시험."특성시험" ("Tab Control") Tap_내구시험."환경설정" ("Tab Control") Tap_내구시험."특성시험" ("Tab Control") Tap_내구시험."그래프" ("Tab Control")] -> w259
          frame "False", Default {
          }
          frame "시험세팅" {
          }
          frame "Main" {
          }
          frame "그래프" {
          }
        }
        n177 = local write "Tab main"(w259) -> ()
      }
      event Value Change {
        n178 = event-data() -> ()  [unwired: 1 in, 1 out]
        n179 = call "fgv_curr-test-info.vi"("cmd"=rw."read") -> ("현재테스트 정보 2"=w268:T24)  [unwired: 10 in]
        n180 = Unbundle By Name(w268) -> ("Ch selection"=w266:T32)
        n181 = call "fgv_rc-config.vi"("cmd"=rw."write", "CapTestConfig"="CapTestConfig") -> ()  [unwired: 9 in, 1 out]
        n182 = Cluster To Array(cluster=w266) -> (array=w270:bool[])
        n183 = call "sub_ch-count.vi"("ch config"=w270) -> ("ch num"=w269:u8)  [unwired: 10 in]
        n184 = call "fgv_curr-test-info.vi"("cmd"=rw."read") -> ("현재테스트 정보 2"=w272:T24)  [unwired: 10 in]
        n185 = Bundle By Name(cluster=w272, "전체채널수"=w269) -> (w271:T24)
        n186 = call "fgv_curr-test-info.vi"("cmd"=rw."write", "현재테스트 정보"=w271) -> ()  [unwired: 9 in, 1 out]
      }
      event "수동_6": Value Change {
        n187 = event-data() -> ()  [unwired: 1 in, 1 out]
        n188 = call "fgv_reg_q.vi"("cmd"=create-rw-close."write", "action"=q-action_reg."Test-Manual") -> ()  [unwired: 8 in, 2 out]
      }
      event "수동_dl950": Value Change {
        n189 = event-data() -> ()  [unwired: 1 in, 6 out]
        n190 = call "fgv_reg_q.vi"("cmd"=create-rw-close."write", "action"=q-action_reg."DL950-Manual") -> ()  [unwired: 8 in, 2 out]
      }
      event Value Change {
        n191 = event-data() -> ()  [unwired: 1 in, 1 out]
        n192 = call "fgv_DL950_config.vi"("cmd"=rw."write", "config"="DL950_config") -> ()  [unwired: 8 in, 2 out]
      }
      event Value Change {
        n193 = event-data() -> ()  [unwired: 1 in, 1 out]
        n194 = call "fgv_rc_breakdonw-specs.vi"("cmd"=rw."write", "BreakdownSpec"="CapTestSpec") -> ()  [unwired: 9 in, 1 out]
      }
      event Timeout {
        n195 = event-data() -> ()  [unwired: 1 in, 1 out]
        n196 = stacked-sequence {
          frame #0 {
            n197 = call "fgv_reg-test_config.vi"("cmd"=rw."read") -> ()  [unwired: 10 in, 1 out]
            n198 = call "fgv_curr-test-info.vi"("cmd"=rw."read") -> ("현재테스트 정보 2"=w299:T24)  [unwired: 10 in]
            n199 = Unbundle By Name(w299) -> ("현재회수"=w285:u32, "테스트 회수"=w292:u32, "전체채널수"=w298:u8, "현재채널번호"=w288:u8)
            "현재 채널" <- w288
            n200 = Divide(x=w292, y=w285) -> (x/y=w293:dbl)
            n201 = Divide(x=w288, y=w298) -> (x/y=w297:dbl)
            n202 = Multiply(x=w293, y=100.0) -> (x*y=→"진행율_채널 %":dbl)
            n203 = Multiply(x=w297, y=100.0) -> (x*y=w290:dbl)
            n204 = Not Equal?(x=w290, y=w290) -> (x != y?=w291:bool)
            n205 = Select(t=0.0, s=w291, f=w290) -> (s? t:f=→"진행율_전체 %":dbl)
          }
          frame #1 {
          }
          frame #2 {
          }
          frame #3 {
            n206 = call "fgv_error.vi"("cmd"=rw."read") -> ("error cluster 2"=→"error cluster 2":T1)  [unwired: 10 in]
          }
        }
      }
      event "cDAQ-9467 Config": Value Change {
        n207 = event-data() -> ()  [unwired: 1 in, 1 out]
        n208 = Concatenate Strings("cDAQ-9467 Config", "/line0:31" ("string")) -> (w305:string)
        n209 = call "fgv_9467_Config.vi"("cmd"=rw."write", "cDAQ-9467 Config"=w305) -> ()  [unwired: 9 in, 1 out]
      }
      event Value Change {
        n210 = event-data() -> ()  [unwired: 1 in, 1 out]
        n211 = call "fgv_9221-config.vi"("cmd"=rw."write", "cDAQ 9221 Config"="cDAQ 9221 Config") -> ()  [unwired: 8 in, 2 out]
      }
      event Value Change {
        n212 = event-data() -> ()  [unwired: 1 in, 1 out]
        n213 = call "fgv_AO_wave-config.vi"("cmd"=rw."write", "Square Wave"="AO_Wave-config") -> ()  [unwired: 9 in, 1 out]
      }
      event Value Change {
        n214 = event-data() -> ()  [unwired: 1 in, 1 out]
        n215 = call "fgv_AO_DAQmx-Config.vi"("cmd"=rw."write", "9269 AO Config"="cDAQ 9269 AO config") -> ()  [unwired: 8 in, 2 out]
      }
      event "TestReset": Value Change {
        n216 = event-data() -> ()  [unwired: 1 in, 1 out]
        n217 = call "fgv_reg_q.vi"("cmd"=create-rw-close."write", "action"=q-action_reg."Test-stop") -> ("error out"=w313:errorcluster)  [unwired: 8 in, 1 out]
        n218 = call "fgv_reg_q.vi"("cmd"=create-rw-close."write", "error in"=w313, "action"=q-action_reg."Test-ini") -> ()  [unwired: 7 in, 2 out]
      }
      event "TestStop": Value Change {
        n219 = event-data() -> ("CtlRef"=w321:refnum<vi>)  [unwired: 1 in]
        n220 = property class="Bool" props=["Label", "Text"](reference=w321) -> ()  [unwired: 1 in, 3 out]
        n221 = call "fgv_reg_q.vi"("cmd"=create-rw-close."read") -> ("error out"=w318:errorcluster, "queue out"=w319:refnum<queue>)  [unwired: 9 in]
        n222 = Flush Queue(queue=w319, error in (no error)=w318) -> ()  [unwired: 3 out]
      }
      event "TestStart": Value Change {
        n223 = event-data() -> ("CtlRef"=w324:refnum<vi>)  [unwired: 1 in]
        n224 = property class="Bool" props=["Label", "Text"](reference=w324) -> ()  [unwired: 1 in, 3 out]
        n225 = call "fgv_reg_q.vi"("cmd"=create-rw-close."write", "action"=q-action_reg."Test-start") -> ()  [unwired: 8 in, 2 out]
      }
      event Value Change {
        n226 = event-data() -> ()  [unwired: 1 in, 1 out]
        n227 = call "fgv_DSP_config.vi"("cmd"=rw."write", "DSP1950 Config"="DSP1950 Config") -> ()  [unwired: 8 in, 2 out]
      }
      event Value Change {
        n228 = event-data() -> ()  [unwired: 1 in, 2 out]
        n229 = call "fgv_4610_config.vi"("cmd"=rw."write", "BP4610 Config"="BP4610 Config") -> ()  [unwired: 8 in, 2 out]
      }
    }
  }
  n230 = flat-sequence {
    tunnel: w1 -> [_]
    frame #0 {
      n231 = call "sub_load-val.vi"("cmd"=enum16{"load", "save"}."save") -> ("error out"=w329:errorcluster)  [unwired: 10 in]
      n232 = call "fgv_params_save-load_cap.vi"("cmd"=T20."LastRUN Save", "error in"=w329) -> ()  [unwired: 8 in, 2 out]
    }
  }
